vi "Set Running.vi"(8 "error in (no error)":errorcluster, 10 "Running":bool, 11 "Panel in":refnum<class "Panel.lvclass">) -> (0 "error out":errorcluster, 3 "Panel out":refnum<class "Panel.lvclass">)   [LabVIEW 2020, in "OOPanel.lvlib" / "Panel.lvclass"]
uses:
  Panel.lvclass
  Panel.lvclass/Panel.ctl
  Visibility State.ctl
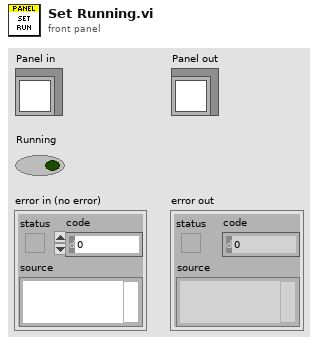
[diagram p1: front panel]
types:
  T1 = typedef "OOPanel.lvlib/Panel.lvclass/Visibility State.ctl" = enum16{"Idle", "Closed", "Hidden", "Visible", "Subpanel"}
  T2 = typedef "OOPanel.lvlib/Panel.lvclass/Ref Data.ctl" = cluster{"Panel Ref":refnum<vi>, "SubPanel":refnum<vi>, "Close":bool, "Running":bool, "State":T1}
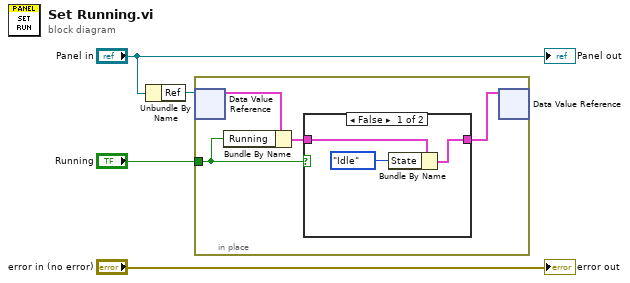
[diagram p0: block diagram]
diagram:
  n1 = Unbundle By Name("Panel in") -> ("Ref"=w3:refnum<data-value>)
  n2 = in-place {
    in-place-border: "Running" -> [w5]
    n3 = in-place-dvr #1(w3) -> (w8:T2)  [unwired: 1 out]
    n4 = Bundle By Name(cluster=w8, "Running"=w5) -> (w7:T2)
    n5 = case shown="False" w5 {
      tunnel: w7 -> [w9 w12]
      tunnel: [w10 w12] -> w6
      frame False {
        n6 = Bundle By Name(cluster=w9, "State"=Visibility_State."Idle") -> (w10:T2)
      }
      frame True {
      }
    }
    n7 = in-place-dvr #1(w6) -> ()  [unwired: 2 out]
  }
  "error out" <- "error in (no error)"
  "Panel out" <- "Panel in"
